vi "PXI_Host_U64_Write_NewMethod_Benchmark.vi"() -> ()   [LabVIEW 2018]
uses:
  <vilib>/Platform/TimedLoop/XDataNode/timing_clust.ctl
  <vilib>/Platform/TimedLoop/XDataNode/nitl_modes.ctl
  <vilib>/Platform/TimedLoop/XDataNode/wakeup.ctl
  cRIO RT/FPGA Bitfile Register Operations/Scalar IO Operations/Write Methods/Write Data Register/Instances/Write U64.vi
  cRIO RT/FPGA Bitfile Register Operations/Scalar IO Operations/Utilities/Find Register Offset.vi
  cRIO RT/FPGA Bitfile Register Operations/Scalar IO Operations/SubVIs/Check Register Data Store.vi
  cRIO RT/FPGA Bitfile Register Operations/Scalar IO Operations/Error Handling/Error 6001.vi
  cRIO RT/FPGA Bitfile Register Operations/Scalar IO Operations/Error Handling/Error 6000.vi
  cRIO RT/FPGA Bitfile Register Operations/Scalar IO Operations/Error Handling/Error 6002.vi
  cRIO RT/FPGA Bitfile Register Operations/Scalar IO Operations/Error Handling/Error 6006.vi
  <vilib>/FPGAPlugInAG/Dynamic/niLvFpga_Close_Dynamic.vi
  <vilib>/platform/TimedLoop/XDataNode/XDataNode.xnode
  <vilib>/rvi/interface/nirviCloseFPGA/nirviCloseFPGA.xnode
  cRIO RT/FPGA Bitfile Register Operations/Scalar IO Operations/FPGA Register IO.lvlib
  <vilib>/Platform/TimedLoop/XDataNode/XDNodeRunTimeDep.lvlib
panel:
  out "Maximum(s)":dbl
  out "Standard deviation":dbl
  out "Waveform Graph":dbl[](graph)
  out "error out":errorcluster
  out "Execution time (s)":dbl
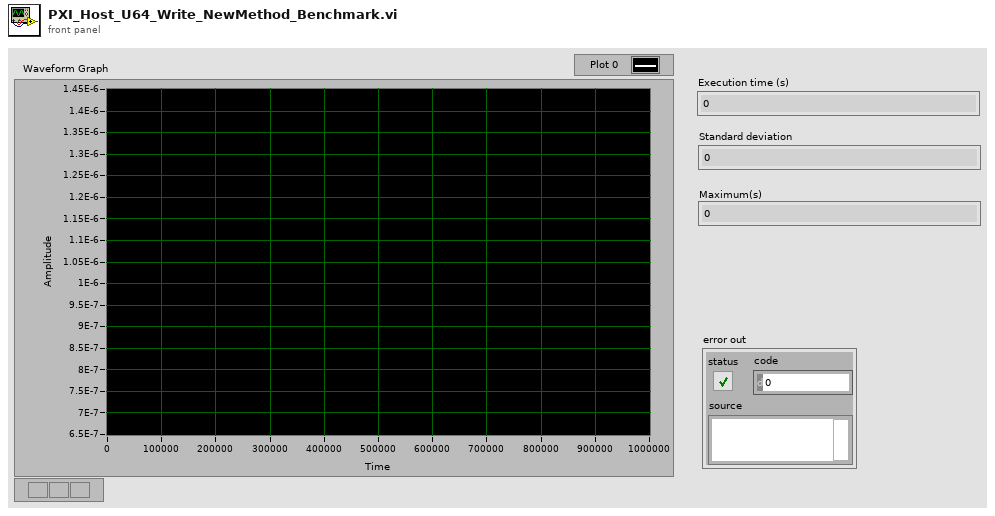
[diagram p1: front panel]
types:
  T1 = typedef "XDNodeRunTimeDep.lvlib/timing_clust.ctl" = cluster{"Expected End [f-1]":u64, "Actual End [f-1]":u64, "Finished Late? [f-1]":bool, "Expected End [i-1]":u64, "Actual End [i-1]":u64, "Finished Late? [i-1]":bool, "Expected Start [i]":u64, "Actual Start [i]":u64, "Expected Start [f]":u64, "Actual Start [f]":u64, "Source Name":string, "Structure Name":string, "Period":i64, "Deadline":i64, "Offset":i64, "Start":i64, "Priority":i32, "Timeout":i32, "Mode":T2, "Wakeup Reason":T3, "Error":errorcluster, "Source Type":string, "Secondary Source Type":string, "Global End Time":u64, "Global Start Time":u64, "Frame Duration":u64, "Iteration Duration":u64, "Assigned CPU":i32, "I/O Scan Engine Mode":u32}
  T2 = typedef "XDNodeRunTimeDep.lvlib/nitl_modes.ctl" = enum32{"No Change", "Process missed periods, maintain original phase", "Discard missed periods, maintain original phase", "Process missed periods, ignore original phase", "Discard missed periods, ignore original phase"}
  T3 = typedef "XDNodeRunTimeDep.lvlib/wakeup.ctl" = enum32{"Normal", "Aborted", "Asynchronous wakeup", "Timing source error", "Timed loop error", "Timeout"}
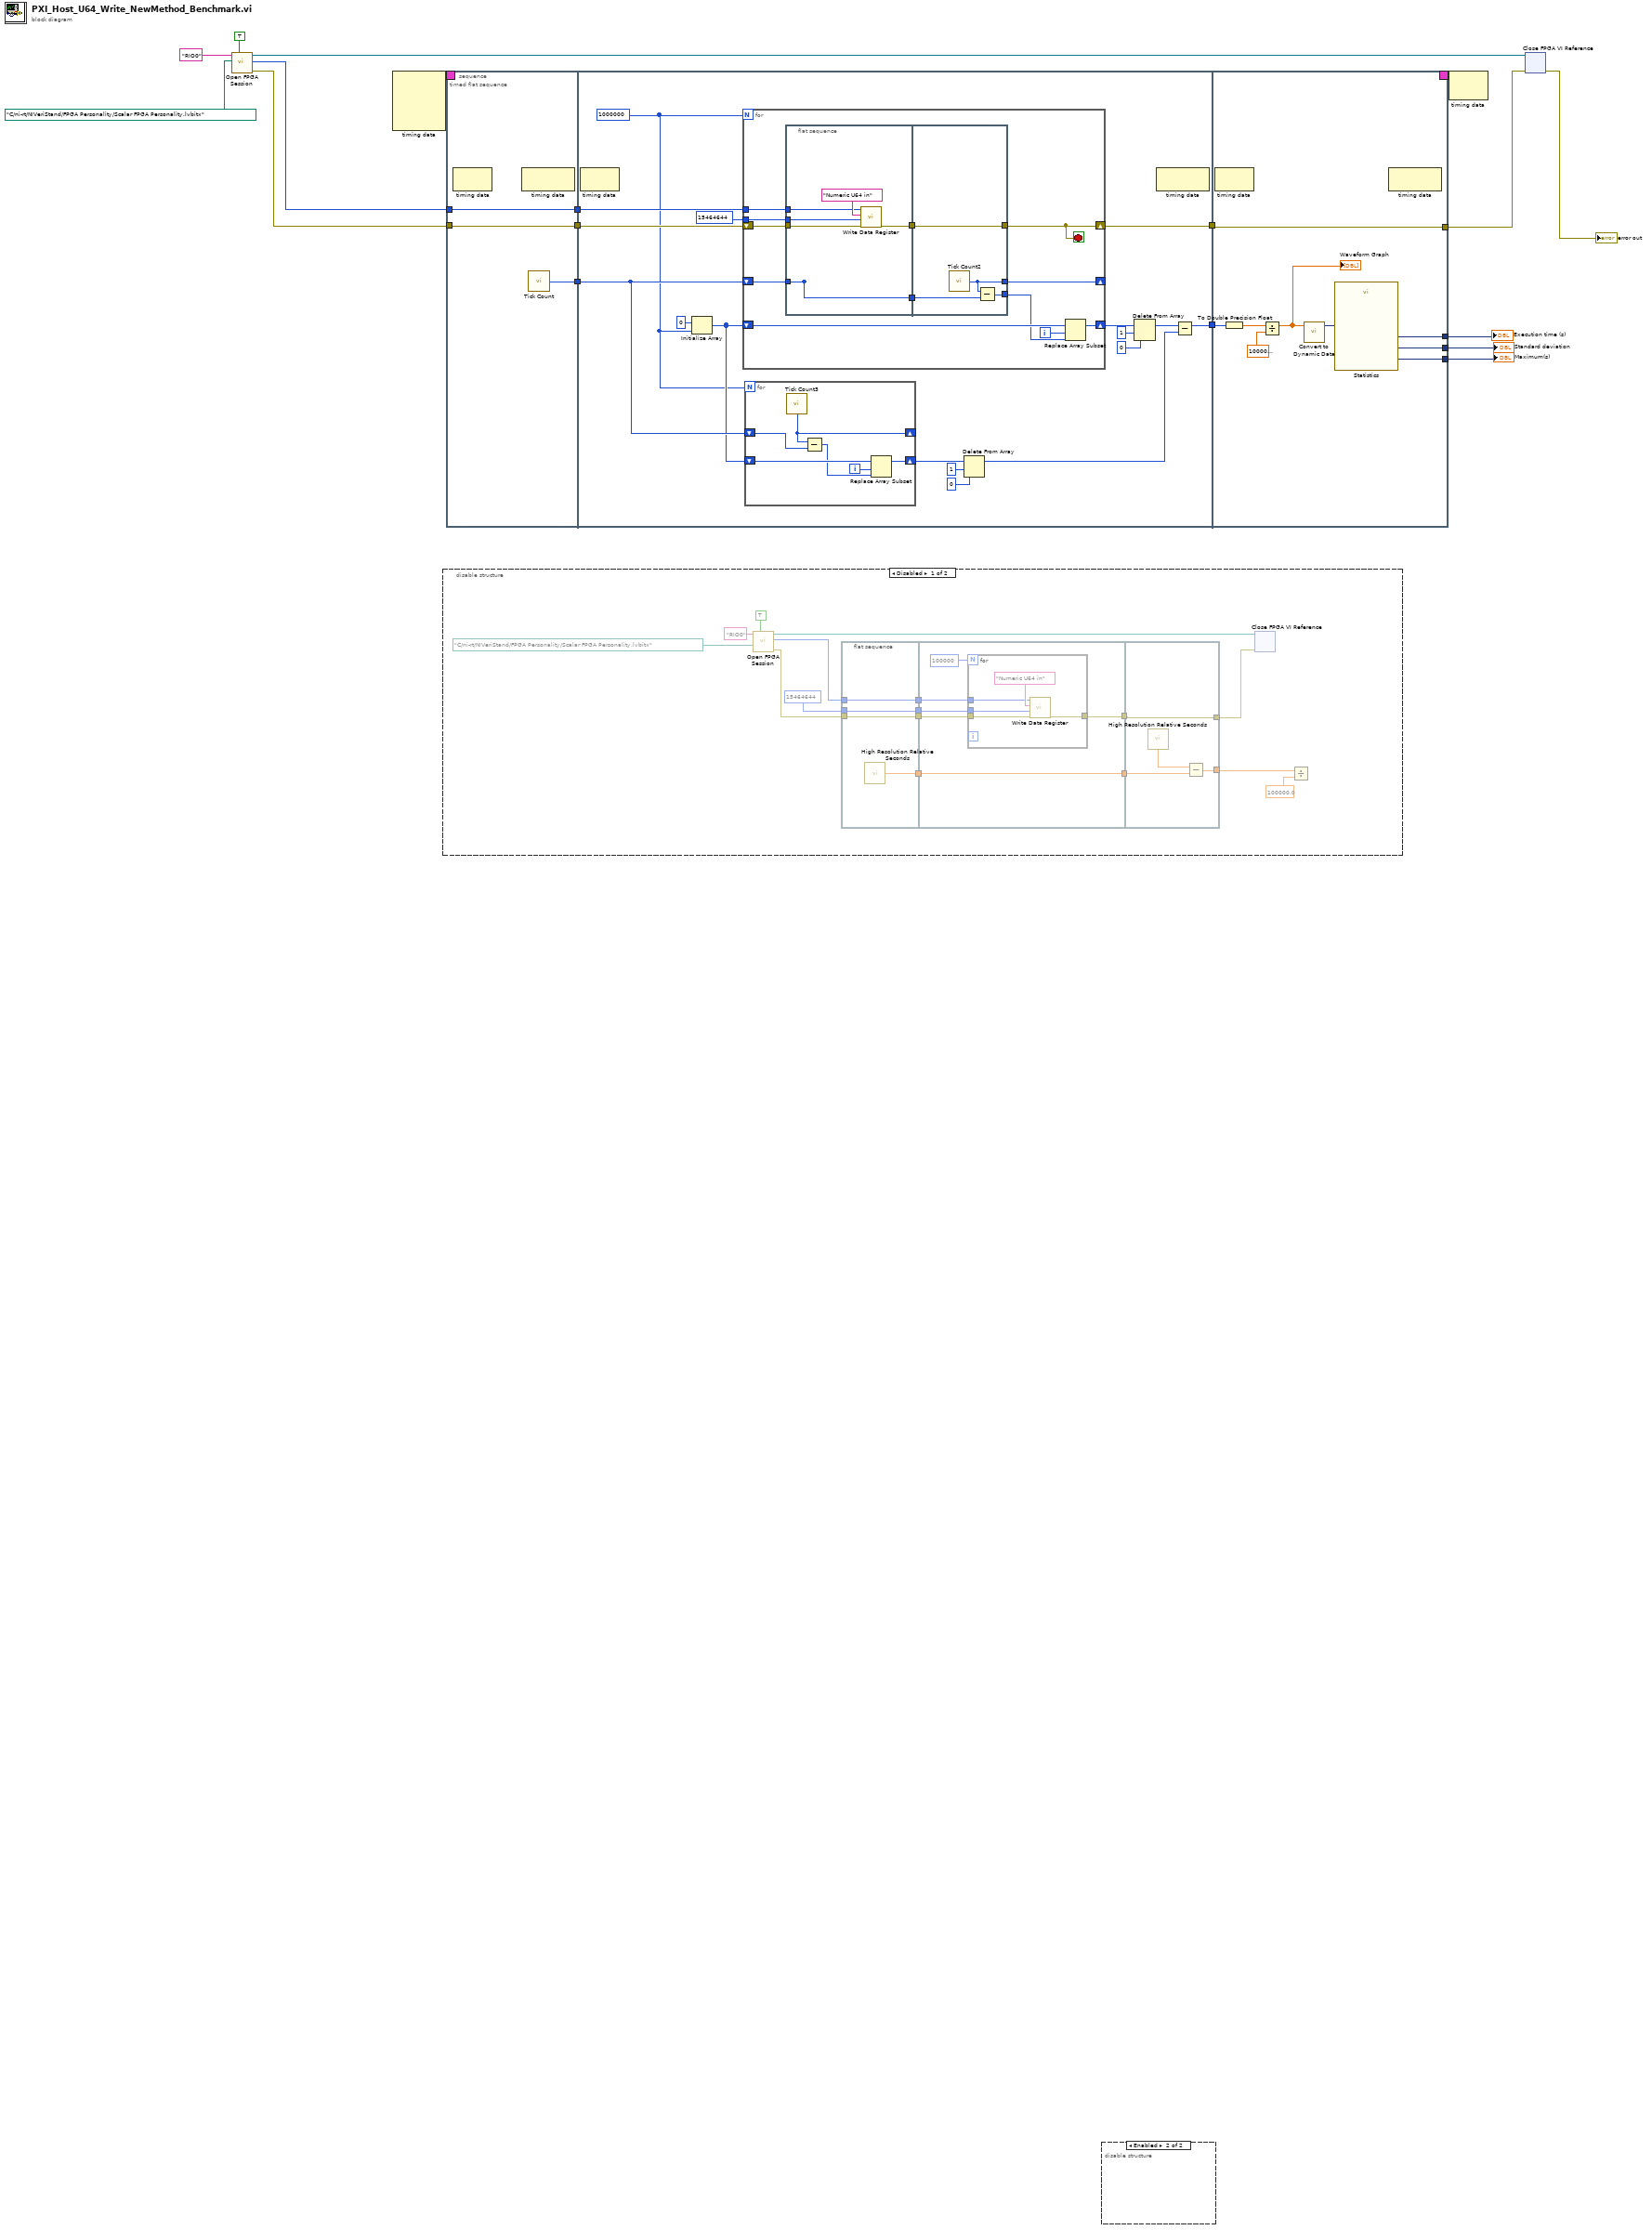
[diagram p0: block diagram]
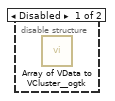
[diagram p3: hidden frame]
diagram:
  n1 = call "Open FPGA Session.vi"("run when loaded (T)"=TRUE, "bitfile path"=path "C:/ni-rt/NIVeriStand/FPGA Personality/Scalar FPGA Personality.lvbitx", "device address"="RIO0") -> ("error out"=w7:errorcluster, "session out"=w11:u32, "bitfile reference out"=w6:refnum<k20>)  [unwired: 6 in]
  n2 = node-c288() -> (w13:T1)  [unwired: 4 in]
  n3 = disable-structure shown="Disabled" {
    frame Disabled {
      n4 = call "Open FPGA Session.vi"("run when loaded (T)"=TRUE, "bitfile path"=path "C:/ni-rt/NIVeriStand/FPGA Personality/Scalar FPGA Personality.lvbitx", "device address"="RIO0") -> ("error out"=w17:errorcluster, "session out"=w21:u32, "bitfile reference out"=w16:refnum<k20>)  [unwired: 6 in]
      n5 = flat-sequence {
        tunnel: [w33] -> w29
        tunnel: w21 -> [w32]
        tunnel: [w32] -> w28
        tunnel: w17 -> [w31]
        tunnel: [w31] -> w27
        tunnel: [w30] -> w26
        tunnel: u64 15464644 ("value in") -> [w30]
        tunnel: [w38] -> w25
        tunnel: w29 -> [w38]
        tunnel: w28 -> [w37]
        tunnel: w27 -> [w36]
        tunnel: [w35] -> w24
        tunnel: w26 -> [w34]
        tunnel: w25 -> [w47]
        tunnel: [w46] -> w23
        tunnel: w24 -> [w45]
        tunnel: [w45] -> w15
        frame #0 {
          n6 = call <vilib>:"High Resolution Relative Seconds.vi"() -> ("relative seconds"=w33:dbl)
        }
        frame #1 {
          n7 = for {
            N: 100000 -> [_]
            tunnel: w37 -> [w41]
            tunnel: w36 -> [w43]
            tunnel: [w44] -> w35
            tunnel: w34 -> [w40]
            n8 = call-poly "Write Data Register.vi"("error in"=w43, "value in"=w40, "register name"="Numeric U64 in", "session in"=w41) -> ("error out"=w44:errorcluster)  [unwired: 6 in, 1 out]
          }
        }
        frame #2 {
          n9 = call <vilib>:"High Resolution Relative Seconds.vi"() -> ("relative seconds"=w48:dbl)
          n10 = Subtract(x=w48, y=w47) -> (x-y=w46:dbl)
        }
      }
      n11 = xnode "Close FPGA VI Reference"("FPGA VI Reference In"=w16, "error in"=w15) -> ()  [unwired: 1 out]
      n12 = Divide(x=w23, y=100000.0) -> ()  [unwired: 1 out]
    }
    frame Enabled {
    }
  }
  n13 = timed-sequence {
    timing: w13 -> [_]
    timing-out: [_] -> w12
    tunnel: w11 -> [w59]
    tunnel: w7 -> [w58]
    tunnel: [w54] -> w5
    tunnel: [w51] -> w3
    tunnel: [w50] -> w2
    tunnel: [w49] -> w1
    n14 = timed-flat-sequence {
      tunnel: w59 -> [w62]
      tunnel: [w62] -> w57
      tunnel: w58 -> [w61]
      tunnel: [w61] -> w56
      tunnel: [w60] -> w53
      tunnel: w57 -> [w81]
      tunnel: w56 -> [w80]
      tunnel: [w79] -> w55
      tunnel: w53 -> [w74]
      tunnel: [w66] -> w52
      tunnel: w55 -> [w120]
      tunnel: [w120] -> w54
      tunnel: w52 -> [w119]
      tunnel: [w117] -> w51
      tunnel: [w114] -> w50
      tunnel: [w113] -> w49
      frame #0 {
        n15 = node-c288() -> ()  [unwired: 1 in, 1 out]
        n16 = node-c288() -> ()  [unwired: 1 in, 1 out]
        n17 = call "Tick Count"() -> ("Tick Count(Ticks)"=w60:u32)
      }
      frame #1 {
        w69 = 1000000
        n18 = node-c288() -> ()  [unwired: 1 in, 1 out]
        n19 = Initialize Array(u32 0, w69) -> (w73:u32[])
        n20 = for {
          N: w69 -> [_]
          tunnel: w81 -> [w100]
          shift-right: [w98] -> _
          shift-left: w74 -> [w97]
          shift-right: [w93] -> w77
          shift-left: w73 -> [w95]
          shift-right: [w91] -> w79
          shift-left: w80 -> [w101]
          tunnel: u64 15464644 ("value in") -> [w90]
          i -> [w92]
          stop <- w91 stop-if-true
          n21 = flat-sequence {
            tunnel: w101 -> [w105]
            tunnel: w100 -> [w103]
            tunnel: [w104] -> w99
            tunnel: [w107] -> _
            tunnel: w97 -> [w107]
            tunnel: [w107] -> w96
            tunnel: w90 -> [w102]
            tunnel: [w111] -> w91
            tunnel: w99 -> [w111]
            tunnel: [w110] -> w98
            tunnel: w96 -> [w109]
            tunnel: [w108] -> w94
            frame #0 {
              n22 = call-poly "Write Data Register.vi"("error in"=w105, "value in"=w102, "register name"="Numeric U64 in", "session in"=w103) -> ("error out"=w104:errorcluster)  [unwired: 6 in, 1 out]
            }
            frame #1 {
              n23 = call "Tick Count2"() -> ("Tick Count(Ticks)"=w110:u32)
              n24 = Subtract(x=w110, y=w109) -> (x-y=w108:u32)
            }
          }
          n25 = Replace Array Subset(array=w95, new element=w94, index=w92) -> (w93:u32[])
        }
        n26 = for {
          N: w69 -> [_]
          shift-right: [w82] -> w70
          shift-left: w73 -> [w85]
          shift-right: [w87] -> _
          shift-left: w74 -> [w86]
          i -> [w83]
          n27 = call "Tick Count3"() -> ("Tick Count(Ticks)"=w87:u32)
          n28 = Subtract(x=w87, y=w86) -> (x-y=w84:u32)
          n29 = Replace Array Subset(array=w85, new element=w84, index=w83) -> (w82:u32[])
        }
        n30 = Delete From Array(array=w70, length=1, index=0) -> (array with subset deleted=w68:u32[])  [unwired: 1 out]
        n31 = Delete From Array(array=w77, length=1, index=0) -> (array with subset deleted=w67:u32[])  [unwired: 1 out]
        n32 = node-c288() -> ()  [unwired: 1 in, 1 out]
        n33 = Subtract(x=w67, y=w68) -> (x-y=w66:u32[])
      }
      frame #2 {
        n34 = node-c288() -> ()  [unwired: 1 in, 1 out]
        n35 = To Double Precision Float(number=w119) -> (double precision float=w116:dbl[])
        n36 = Divide(x=w116, y=1000000000.0) -> (x/y=w112:dbl[])
        "Waveform Graph" <- w112
        n37 = call "Convert to Dynamic Data"("Array"=w112) -> ("Dynamic Data Type"=w118:dynamicdata)  [unwired: 3 in]
        n38 = call "Statistics"("Signals"=w118) -> ("Standard Dev"=w114:dynamicdata, "Arithmetic Mean"=w117:dynamicdata, "Maximum"=w113:dynamicdata)  [unwired: 23 in, 1 out]
        n39 = node-c288() -> ()  [unwired: 1 in, 1 out]
      }
    }
  }
  "Execution time (s)" <- w3
  "Standard deviation" <- w2
  "Maximum(s)" <- w1
  n40 = disable-structure shown="Enabled" {
    frame Disabled {
      n41 = call <userlib>:"Array of VData to VCluster__ogtk.vi"() -> ()  [unwired: 10 in, 2 out]
    }
    frame Enabled {
    }
  }
  n42 = node-c288(w12) -> ()  [unwired: 1 out]
  n43 = xnode "Close FPGA VI Reference"("FPGA VI Reference In"=w6, "error in"=w5) -> ("error out"=→"error out":errorcluster)
